vi "initialize.vi"(8 "error in (no error)":errorcluster, 10 "bitrate":T1, 11 "channel handle":u16 format="%x") -> (0 "error out":errorcluster)   [LabVIEW 2024, in "atsj peakcan basic.lvlib"]
doc: "Initializes a PCAN bus (channel).\n\nCopyright (c) 2025 ATSJ (www.atsj.eu)"
uses:
  atsj peakcan basic.lvlib
  bitrate.ctl
  support/x64/PCANBasic.dll
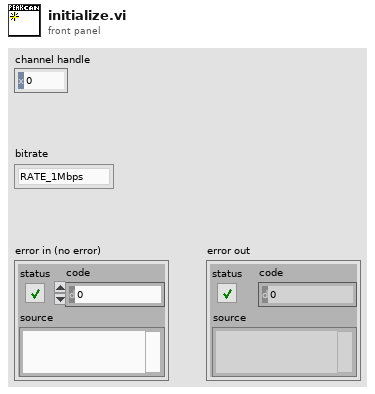
[diagram p1: front panel]
types:
  T1 = typedef "atsj peakcan basic.lvlib/bitrate.ctl" = enum16{"RATE_1Mbps", "RATE_800kbps", "RATE_500kbps", "RATE_250kbps", "RATE_125kbps", "RATE_100kbps", "RATE_95kbps", "RATE_83kbps", "RATE_50kbps", "RATE_47kbps", "RATE_33kbps", "RATE_20kbps", "RATE_10kbps", "RATE_5kbps"}
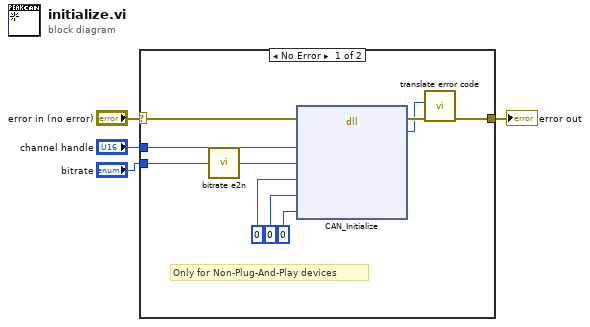
[diagram p0: block diagram]
diagram:
  n1 = case shown="No Error" "error in (no error)" {
    selector: "error in (no error)" -> [w11 w15]
    tunnel: [w6 w15] -> w3
    tunnel: "channel handle" -> [w10 _]
    tunnel: "bitrate" -> [w9 _]
    frame No Error {
      # "Only for Non-Plug-And-Play devices"
      n2 = call "bitrate e2n.vi"("enum"=w9) -> ("number"=w8:u16)
      n3 = dll-call lib="C:/atsj/plateau/atsj-peakcan-basic-for-labview/src/support/x64/PCANBasic.dll" fn="CAN_Initialize"(error in=w11, "Channel"=w10, "Btr0Btr1"=w8, "HwType"=u8 0, "IOPort"=u32 0, "Interrupt"=u16 0) -> (error out=w7:errorcluster, "Status"=w5:u32)  [unwired: 7 in, 1 out]
      n4 = call "translate error code.vi"("error in (no error)"=w7, "error code"=w5) -> ("error out"=w6:errorcluster)  [unwired: 9 in]
    }
    frame Error {
    }
  }
  "error out" <- w3
